vi "SquareSpiral.vi"(1 "Height":dbl, 2 "Width":dbl, 3 "Iteration Number":u16, 4 "SpiralThickness (0 to 1)":dbl) -> (0 "ProjectorCoordinates":cluster{"X":dbl, "Y":dbl}[](array[cluster]))   [LabVIEW 2019]
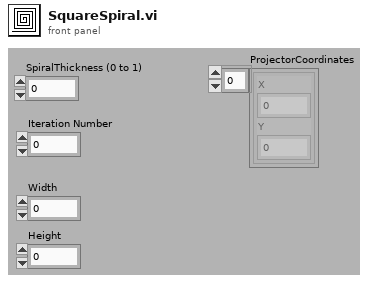
[diagram p1: front panel]
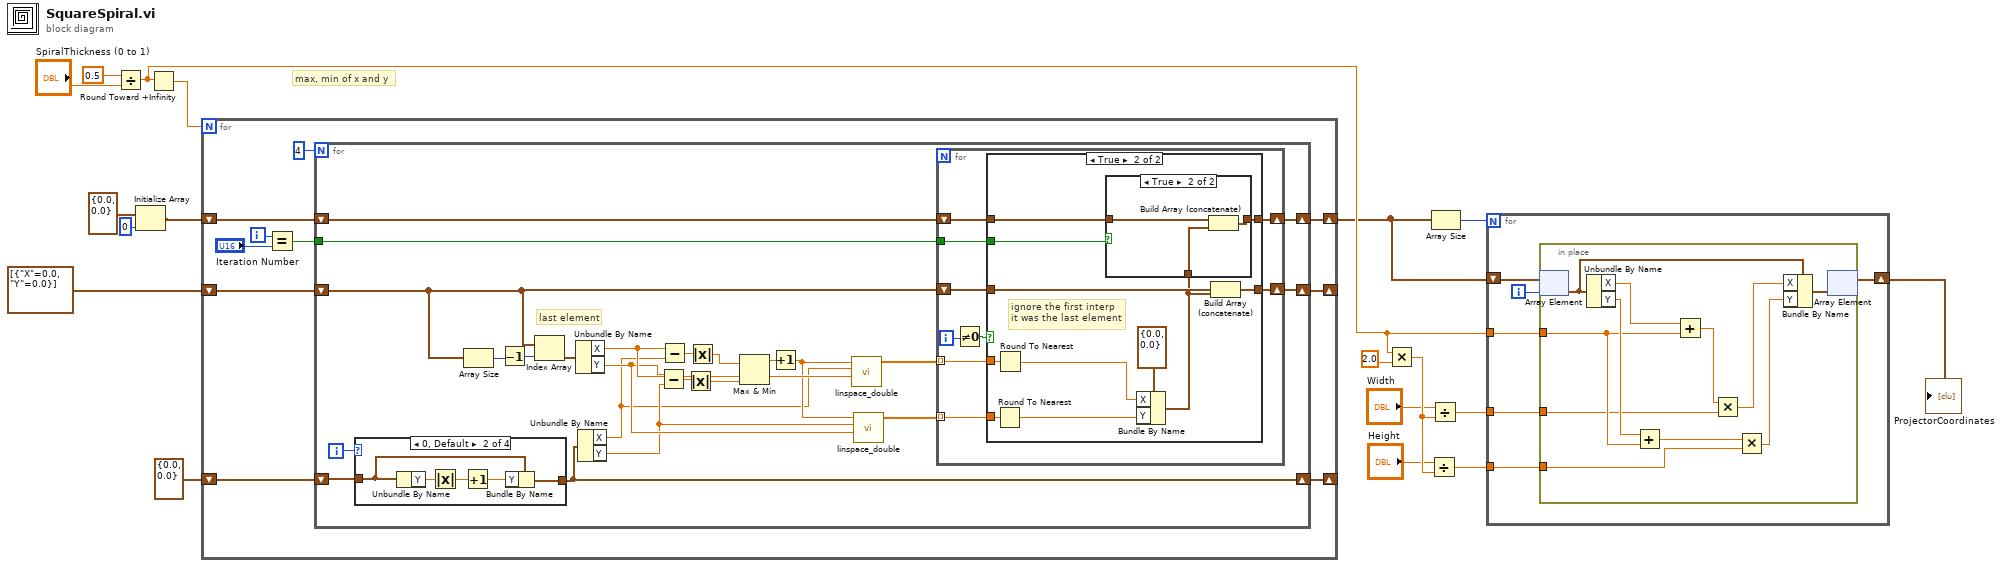
[diagram p0: block diagram]
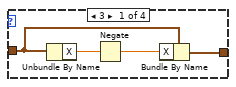
[diagram p2: hidden frame]
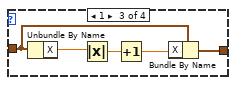
[diagram p3: hidden frame]
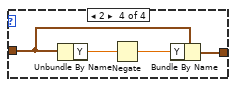
[diagram p4: hidden frame]
diagram:
  # "max, min of x and y"
  n1 = Divide(x=0.5, y="SpiralThickness (0 to 1)") -> (x/y=w8:dbl)
  n2 = Initialize Array(cluster{"X":dbl, "Y":dbl} {"X"=0.0, "Y"=0.0}, 0) -> (w3:cluster{"X":dbl, "Y":dbl}[])
  n3 = Round Toward +Infinity(x=w8) -> (ceil(x): smallest int >= x=w6:dbl)
  n4 = for {
    N: w6 -> [_]
    shift-right: [w26] -> _
    shift-left: cluster{"X":dbl, "Y":dbl}[] [{"X"=0.0, "Y"=0.0}] ("XY Graph") -> [w28]
    shift-right: [w24] -> _
    shift-left: cluster{"X":dbl, "Y":dbl} {"X"=0.0, "Y"=0.0} -> [w27]
    shift-right: [w19] -> w4
    shift-left: w3 -> [w20]
    i -> [w23]
    n5 = Equal?(x=w23, y="Iteration Number") -> (x = y?=w21:bool)
    n6 = for {
      N: u16 4 -> [_]
      shift-right: [w45] -> w26
      shift-left: w28 -> [w37]
      shift-right: [w40] -> w24
      shift-left: w27 -> [w41]
      tunnel: w21 -> [w31]
      shift-right: [w30] -> w19
      shift-left: w20 -> [w32]
      i -> [w29]
      # "last element"
      n7 = case shown="0, Default" w29 {
        tunnel: w41 -> [w55 w57 w65 w67]
        tunnel: [w54 w56 w64 w66] -> w40
        frame 3 {
          n8 = Unbundle By Name(w55) -> ("X"=w52:dbl)
          n9 = Negate(x=w52) -> (-x=w53:dbl)
          n10 = Bundle By Name(cluster=w55, "X"=w53) -> (w54:cluster{"X":dbl, "Y":dbl})
        }
        frame 0, Default {
          n11 = Unbundle By Name(w57) -> ("Y"=w60:dbl)
          n12 = Absolute Value(x=w60) -> (abs(x)=w59:dbl)
          n13 = Increment(x=w59) -> (x+1=w58:dbl)
          n14 = Bundle By Name(cluster=w57, "Y"=w58) -> (w56:cluster{"X":dbl, "Y":dbl})
        }
        frame 1 {
          n15 = Unbundle By Name(w65) -> ("X"=w61:dbl)
          n16 = Absolute Value(x=w61) -> (abs(x)=w63:dbl)
          n17 = Increment(x=w63) -> (x+1=w62:dbl)
          n18 = Bundle By Name(cluster=w65, "X"=w62) -> (w64:cluster{"X":dbl, "Y":dbl})
        }
        frame 2 {
          n19 = Unbundle By Name(w67) -> ("Y"=w69:dbl)
          n20 = Negate(x=w69) -> (-x=w68:dbl)
          n21 = Bundle By Name(cluster=w67, "Y"=w68) -> (w66:cluster{"X":dbl, "Y":dbl})
        }
      }
      n22 = Array Size(array=w37) -> (size(s)=w34:i32)
      n23 = Decrement(x=w34) -> (x-1=w33:i32)
      n24 = Index Array(array=w37, index=w33) -> (element=w35:cluster{"X":dbl, "Y":dbl})
      n25 = Unbundle By Name(w35) -> ("X"=w48:dbl, "Y"=w47:dbl)
      n26 = Unbundle By Name(w40) -> ("X"=w38:dbl, "Y"=w39:dbl)
      n27 = Subtract(x=w47, y=w39) -> (x-y=w50:dbl)
      n28 = Subtract(x=w48, y=w38) -> (x-y=w51:dbl)
      n29 = Absolute Value(x=w50) -> (abs(x)=w36:dbl)
      n30 = Absolute Value(x=w51) -> (abs(x)=w49:dbl)
      n31 = Max & Min(x=w49, y=w36) -> (max(x,y)=w43:dbl)  [unwired: 1 out]
      n32 = Increment(x=w43) -> (x+1=w42:dbl)
      n33 = call "linspace_double.vi"("start"=w48, "end"=w38, "samples"=w42) -> ("Ramp Pattern"=w44:dbl[])  [unwired: 8 in]
      n34 = call "linspace_double.vi"("start"=w47, "end"=w39, "samples"=w42) -> ("Ramp Pattern"=w46:dbl[])  [unwired: 8 in]
      n35 = for {
        tunnel: w44 -> [w75] mode=indexing
        tunnel: w46 -> [w77] mode=indexing
        shift-right: [w76] -> w45
        shift-left: w37 -> [w78]
        shift-right: [w70] -> w30
        shift-left: w32 -> [w71]
        tunnel: w31 -> [w72]
        i -> [w74]
        n36 = Not Equal To 0?(x=w74) -> (x != 0?=w73:bool)
        n37 = case shown="True" w73 {
          tunnel: w78 -> [w80 w91]
          tunnel: w77 -> [_ w90]
          tunnel: [w80 w89] -> w76
          tunnel: w75 -> [_ w88]
          tunnel: w72 -> [_ w84]
          tunnel: w71 -> [w79 w83]
          tunnel: [w79 w81] -> w70
          frame False {
          }
          frame True {
            # "ignore the first interp\nit was the last element"
            n38 = Round To Nearest(number=w90) -> (nearest integer value=w85:dbl)
            n39 = Round To Nearest(number=w88) -> (nearest integer value=w86:dbl)
            n40 = Bundle By Name(cluster=cluster{"X":dbl, "Y":dbl} {"X"=0.0, "Y"=0.0}, "X"=w86, "Y"=w85) -> (w82:cluster{"X":dbl, "Y":dbl})
            n41 = case shown="True" w84 {
              tunnel: w83 -> [w92 w94]
              tunnel: w82 -> [_ w95]
              tunnel: [w92 w93] -> w81
              frame False {
              }
              frame True {
                n42 = Build Array (concatenate)(w94, w95) -> (w93:cluster{"X":dbl, "Y":dbl}[])
              }
            }
            n43 = Build Array (concatenate)(w91, w82) -> (w89:cluster{"X":dbl, "Y":dbl}[])
          }
        }
      }
    }
  }
  n44 = Multiply(x=w8, y=2.0) -> (x*y=w13:dbl)
  n45 = Divide(x="Height", y=w13) -> (x/y=w10:dbl)
  n46 = Divide(x="Width", y=w13) -> (x/y=w9:dbl)
  n47 = Array Size(array=w4) -> (size(s)=w17:i32)
  n48 = for {
    N: w17 -> [_]
    shift-right: [w99] -> w14
    shift-left: w4 -> [w101]
    tunnel: w8 -> [w98]
    tunnel: w10 -> [w97]
    tunnel: w9 -> [w96]
    i -> [w100]
    n49 = in-place {
      in-place-border: w98 -> [w108]
      in-place-border: w97 -> [w104]
      in-place-border: w96 -> [w106]
      n50 = in-place-array #1(w101, w100) -> (w111:cluster{"X":dbl, "Y":dbl})
      n51 = Unbundle By Name(w111) -> ("X"=w110:dbl, "Y"=w109:dbl)
      n52 = Add(x=w109, y=w108) -> (x+y=w105:dbl)
      n53 = Add(x=w110, y=w108) -> (x+y=w107:dbl)
      n54 = Multiply(x=w107, y=w106) -> (x*y=w102:dbl)
      n55 = Multiply(x=w105, y=w104) -> (x*y=w103:dbl)
      n56 = Bundle By Name(cluster=w111, "X"=w102, "Y"=w103) -> (w112:cluster{"X":dbl, "Y":dbl})
      n57 = in-place-array #1(w112) -> (w99:cluster{"X":dbl, "Y":dbl}[])  [unwired: 1 out]
    }
  }
  "ProjectorCoordinates" <- w14
